vi "processamento_ultrassonico.vi"() -> ()   [LabVIEW 2022 SP3]
uses:
  <vilib>/Analysis/baseanly.llb/Mean (DBL).vi
  <vilib>/Analysis/NI_AALBase.lvlib
panel:
  out "Waveform Graph 2":dbl[][](graph)
  out "appended array 2":dbl[][](array[numeric])
  out "mean 3":dbl format="%0.2f"
  out "com_objeto_maior_trat_2":dbl[](graph)
  out "mean 2":dbl format="%0.2f"
  out "com_peca_trat_2":dbl[](graph)
  out "array":dbl[](array[numeric])
  out "mean":dbl format="%0.2f"
  out "sem_objeto_trat 2":dbl[](graph)
  out "Waveform Graph":dbl[][](graph)
  out "appended array":dbl[][](array[numeric])
  out "mean_com_objeto_maior":dbl format="%0.2f"
  out "com_objeto_maior_trat":dbl[](graph)
  out "direito 3":dbl
  out "esquerdo 3":dbl
  out "mean_com_peca":dbl format="%0.2f"
  out "com_peca_trat":dbl[](graph)
  out "direito 2":dbl
  out "esquerdo 2":dbl
  in  "com_objeto_maior":path
  in  "com_peca":path
  out "com_objeto_maior":dbl[](graph)
  out "com_peca":dbl[](graph)
  out "mean_sem_objeto":dbl format="%0.2f"
  out "sem_objeto_trat":dbl[](graph)
  in  "stop":bool
  out "direito":dbl
  out "esquerdo":dbl
  out "sem_objeto":dbl[](graph)
  in  "sem objeto":path
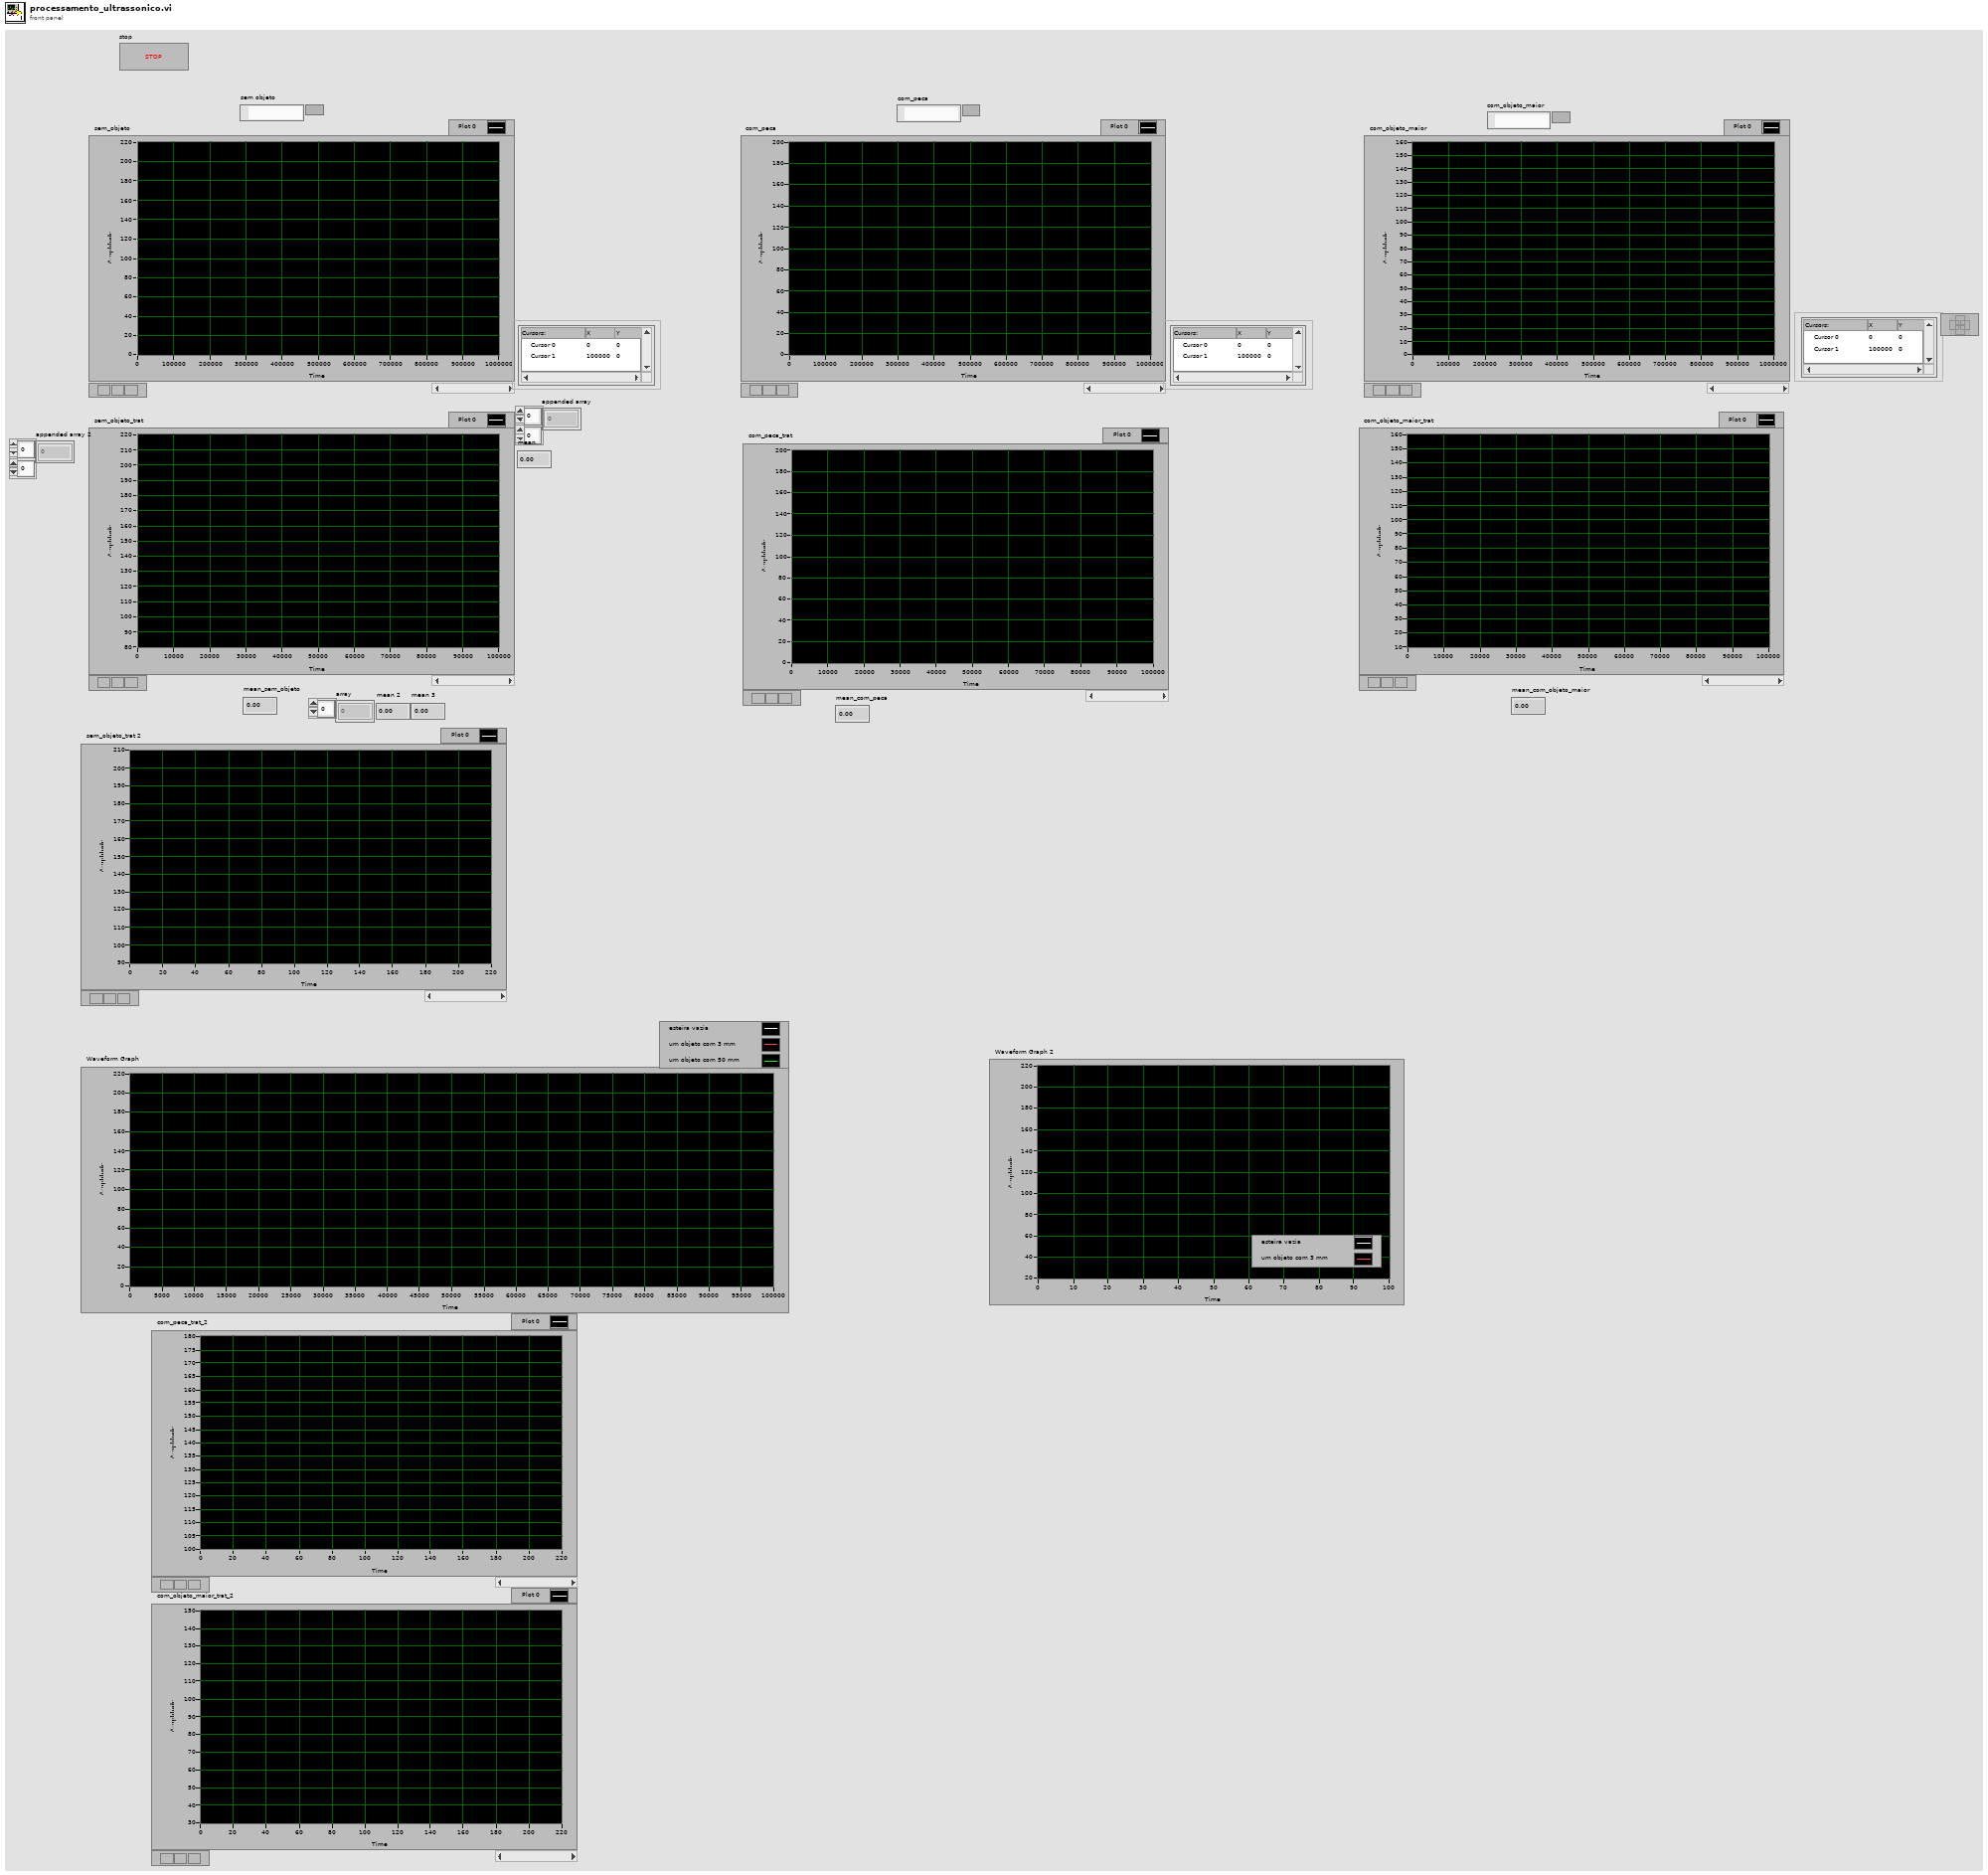
[diagram p1: front panel]
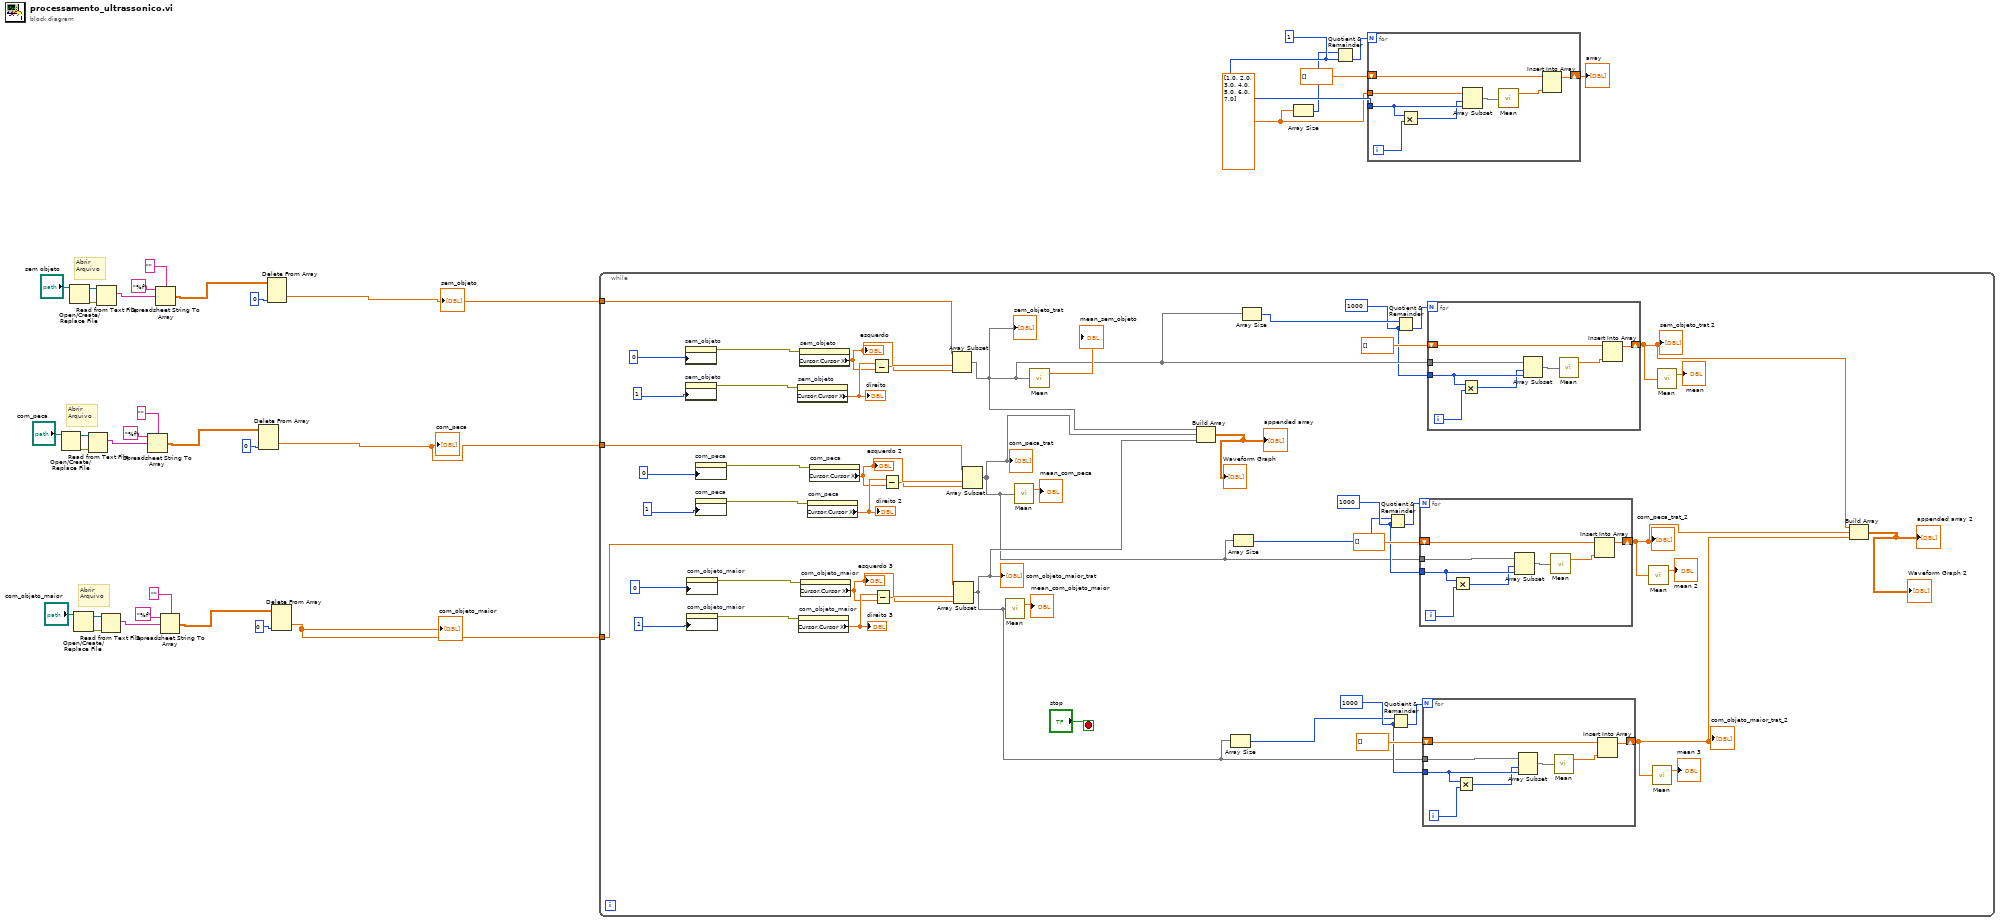
[diagram p0: block diagram]
diagram:
  w3 = dbl[] [1.0, 2.0, 3.0, 4.0, 5.0, 6.0, 7.0]
  w4 = 1
  # "Abrir \nArquivo"
  # "Abrir \nArquivo"
  # "Abrir \nArquivo"
  n1 = Open/Create/Replace File(file path (use dialog)="com_peca") -> (refnum out=w24:refnum<file>, error out=w22:errorcluster)  [unwired: 5 in, 1 out]
  n2 = Open/Create/Replace File(file path (use dialog)="sem objeto") -> (refnum out=w33:refnum<file>, error out=w31:errorcluster)  [unwired: 5 in, 1 out]
  n3 = Open/Create/Replace File(file path (use dialog)="com_objeto_maior") -> (refnum out=w16:refnum<file>, error out=w14:errorcluster)  [unwired: 5 in, 1 out]
  n4 = Read from Text File(file (use dialog)=w24, error in=w22) -> (text=w21:string)  [unwired: 2 in, 3 out]
  n5 = Read from Text File(file (use dialog)=w33, error in=w31) -> (text=w30:string)  [unwired: 2 in, 3 out]
  n6 = Read from Text File(file (use dialog)=w16, error in=w14) -> (text=w13:string)  [unwired: 2 in, 3 out]
  n7 = Spreadsheet String To Array(delimiter (Tab)="", format string="%f", spreadsheet string=w21) -> (array=w17:dbl[][])  [unwired: 1 in]
  n8 = Spreadsheet String To Array(delimiter (Tab)="", format string="%f", spreadsheet string=w30) -> (array=w26:dbl[][])  [unwired: 1 in]
  n9 = Spreadsheet String To Array(delimiter (Tab)="", format string="%f", spreadsheet string=w13) -> (array=w9:dbl[][])  [unwired: 1 in]
  n10 = Delete From Array(array=w17, index (col)=0 ("disabled index (col)")) -> (deleted portion=w8:dbl[])  [unwired: 2 in, 1 out]
  "com_peca" <- w8
  n11 = Delete From Array(array=w26, index (col)=0 ("disabled index (col)")) -> (deleted portion=w25:dbl[])  [unwired: 2 in, 1 out]
  "sem_objeto" <- w25
  n12 = Delete From Array(array=w9, index (col)=0 ("disabled index (col)")) -> (deleted portion=w7:dbl[])  [unwired: 2 in, 1 out]
  "com_objeto_maior" <- w7
  n13 = while {
    tunnel: w25 -> [w75]
    tunnel: w8 -> [w59]
    tunnel: w7 -> [w58]
    stop <- "stop" stop-if-true
    w42 = 1000
    w46 = 1000
    w50 = 1000
    n14 = property on="sem_objeto" class="WFGraph (strict)"("Active Cursor"=u32 0) -> (error out=w84:errorcluster)  [unwired: 2 in, 1 out]
    n15 = property on="sem_objeto" class="WFGraph (strict)"("Active Cursor"=u32 1) -> (error out=w82:errorcluster)  [unwired: 2 in, 1 out]
    n16 = property on="com_objeto_maior" class="WFGraph (strict)"("Active Cursor"=u32 0) -> (error out=w67:errorcluster)  [unwired: 2 in, 1 out]
    n17 = property on="com_objeto_maior" class="WFGraph (strict)"("Active Cursor"=u32 1) -> (error out=w65:errorcluster)  [unwired: 2 in, 1 out]
    n18 = property on="com_peca" class="WFGraph (strict)"("Active Cursor"=u32 0) -> (error out=w74:errorcluster)  [unwired: 2 in, 1 out]
    n19 = property on="com_peca" class="WFGraph (strict)"("Active Cursor"=u32 1) -> (error out=w73:errorcluster)  [unwired: 2 in, 1 out]
    n20 = property on="sem_objeto" class="WFGraph (strict)"(error in=w82) -> ("Cursor.Cursor X"=w80:dbl)  [unwired: 1 in, 2 out]
    "direito" <- w80
    n21 = property on="com_objeto_maior" class="WFGraph (strict)"(error in=w65) -> ("Cursor.Cursor X"=w63:dbl)  [unwired: 1 in, 2 out]
    "direito 3" <- w63
    n22 = property on="sem_objeto" class="WFGraph (strict)"(error in=w84) -> ("Cursor.Cursor X"=w78:dbl)  [unwired: 1 in, 2 out]
    "esquerdo" <- w78
    n23 = property on="com_objeto_maior" class="WFGraph (strict)"(error in=w67) -> ("Cursor.Cursor X"=w62:dbl)  [unwired: 1 in, 2 out]
    "esquerdo 3" <- w62
    n24 = property on="com_peca" class="WFGraph (strict)"(error in=w73) -> ("Cursor.Cursor X"=w71:dbl)  [unwired: 1 in, 2 out]
    "direito 2" <- w71
    n25 = property on="com_peca" class="WFGraph (strict)"(error in=w74) -> ("Cursor.Cursor X"=w70:dbl)  [unwired: 1 in, 2 out]
    "esquerdo 2" <- w70
    n26 = Subtract(x=w80, y=w78) -> (x-y=w77:dbl)
    n27 = Subtract(x=w63, y=w62) -> (x-y=w61:dbl)
    n28 = Subtract(x=w71, y=w70) -> (x-y=w69:dbl)
    n29 = Array Subset(array=w75, index=w78, length=w77) -> (w55:dbl[])
    "sem_objeto_trat" <- w55
    n30 = Array Subset(array=w58, index=w62, length=w61) -> (w39:dbl[])
    "com_objeto_maior_trat" <- w39
    n31 = Array Subset(array=w59, index=w70, length=w69) -> (w38:dbl[])
    "com_peca_trat" <- w38
    n32 = call-poly <vilib>:"Mean.vi"("X"=w39) -> ("mean"=→"mean_com_objeto_maior":dbl)  [unwired: 1 out]
    n33 = call-poly <vilib>:"Mean.vi"("X"=w38) -> ("mean"=→"mean_com_peca":dbl)  [unwired: 1 out]
    n34 = call-poly <vilib>:"Mean.vi"("X"=w55) -> ("mean"=→"mean_sem_objeto":dbl)  [unwired: 1 out]
    n35 = Build Array(w55, w38, w39) -> (→"appended array" →"Waveform Graph":dbl[][])
    n36 = Array Size(array=w39) -> (size(s)=w40:i32)
    n37 = Array Size(array=w38) -> (size(s)=w41:i32)
    n38 = Array Size(array=w55) -> (size(s)=w54:i32)
    n39 = Quotient & Remainder(x=w41, y=w46) -> (floor(x/y)=w49:i32)  [unwired: 1 out]
    n40 = Quotient & Remainder(x=w40, y=w42) -> (floor(x/y)=w45:i32)  [unwired: 1 out]
    n41 = Quotient & Remainder(x=w54, y=w50) -> (floor(x/y)=w53:i32)  [unwired: 1 out]
    n42 = for {
      N: w49 -> [_]
      tunnel: w38 -> [w100]
      tunnel: w46 -> [w99]
      shift-right: [w93] -> w35
      shift-left: dbl[] [] ("array") -> [w95]
      i -> [w98]
      n43 = Multiply(x=w99, y=w98) -> (x*y=w97:i32)
      n44 = Array Subset(array=w100, index=w97, length=w99) -> (w96:dbl[])
      n45 = call-poly <vilib>:"Mean.vi"("X"=w96) -> ("mean"=w94:dbl)  [unwired: 1 out]
      n46 = Insert Into Array(array=w95, new element=w94) -> (w93:dbl[])  [unwired: 1 in]
    }
    "com_peca_trat_2" <- w35
    n47 = for {
      N: w45 -> [_]
      tunnel: w39 -> [w92]
      tunnel: w42 -> [w91]
      shift-right: [w85] -> w34
      shift-left: dbl[] [] ("array") -> [w87]
      i -> [w90]
      n48 = Multiply(x=w91, y=w90) -> (x*y=w89:i32)
      n49 = Array Subset(array=w92, index=w89, length=w91) -> (w88:dbl[])
      n50 = call-poly <vilib>:"Mean.vi"("X"=w88) -> ("mean"=w86:dbl)  [unwired: 1 out]
      n51 = Insert Into Array(array=w87, new element=w86) -> (w85:dbl[])  [unwired: 1 in]
    }
    "com_objeto_maior_trat_2" <- w34
    n52 = for {
      N: w53 -> [_]
      tunnel: w55 -> [w108]
      tunnel: w50 -> [w107]
      shift-right: [w101] -> w36
      shift-left: dbl[] [] ("array") -> [w103]
      i -> [w106]
      n53 = Multiply(x=w107, y=w106) -> (x*y=w105:i32)
      n54 = Array Subset(array=w108, index=w105, length=w107) -> (w104:dbl[])
      n55 = call-poly <vilib>:"Mean.vi"("X"=w104) -> ("mean"=w102:dbl)  [unwired: 1 out]
      n56 = Insert Into Array(array=w103, new element=w102) -> (w101:dbl[])  [unwired: 1 in]
    }
    "sem_objeto_trat 2" <- w36
    n57 = call-poly <vilib>:"Mean.vi"("X"=w35) -> ("mean"=→"mean 2":dbl)  [unwired: 1 out]
    n58 = call-poly <vilib>:"Mean.vi"("X"=w34) -> ("mean"=→"mean 3":dbl)  [unwired: 1 out]
    n59 = call-poly <vilib>:"Mean.vi"("X"=w36) -> ("mean"=→"mean":dbl)  [unwired: 1 out]
    n60 = Build Array(w36, w35, w34) -> (→"appended array 2" →"Waveform Graph 2":dbl[][])
  }
  n61 = Array Size(array=w3) -> (size(s)=w2:i32)
  n62 = Quotient & Remainder(x=w2, y=w4) -> (floor(x/y)=w6:i32)  [unwired: 1 out]
  n63 = for {
    N: w6 -> [_]
    tunnel: w3 -> [w116]
    tunnel: w4 -> [w115]
    shift-right: [w109] -> w1
    shift-left: dbl[] [] ("array") -> [w111]
    i -> [w114]
    n64 = Multiply(x=w115, y=w114) -> (x*y=w113:i32)
    n65 = Array Subset(array=w116, index=w113, length=w115) -> (w112:dbl[])
    n66 = call-poly <vilib>:"Mean.vi"("X"=w112) -> ("mean"=w110:dbl)  [unwired: 1 out]
    n67 = Insert Into Array(array=w111, new element=w110) -> (w109:dbl[])  [unwired: 1 in]
  }
  "array" <- w1
